vi "Boolean Check Output Result.vi"(9 "Output Value in":cluster{"Name":string, "Variant Data":variant}, 10 "Step Output in":T5, 11 "Execution in":refnum<data-value>) -> (2 "Measure Result out":T1, 3 "Execution out":refnum<data-value>)   [LabVIEW 2015, in "Execution.lvclass"]
uses:
  Execution.lvclass
  Step/STEP_OUTPUT.ctl
  Step/OUTPUT_DATA_TYPE.ctl
  OutputUI/OUTPUT_CHECK_TYPE.ctl
  Step/OUTPUT_VALUE_TYPE.ctl
  STEP_MEASURE_RESULT.ctl
  Step/STEP_STATUS.ctl
  <vilib>/Utility/error.llb/DialogType.ctl
  Get Limit Value Boolean.vi
  Step.lvclass
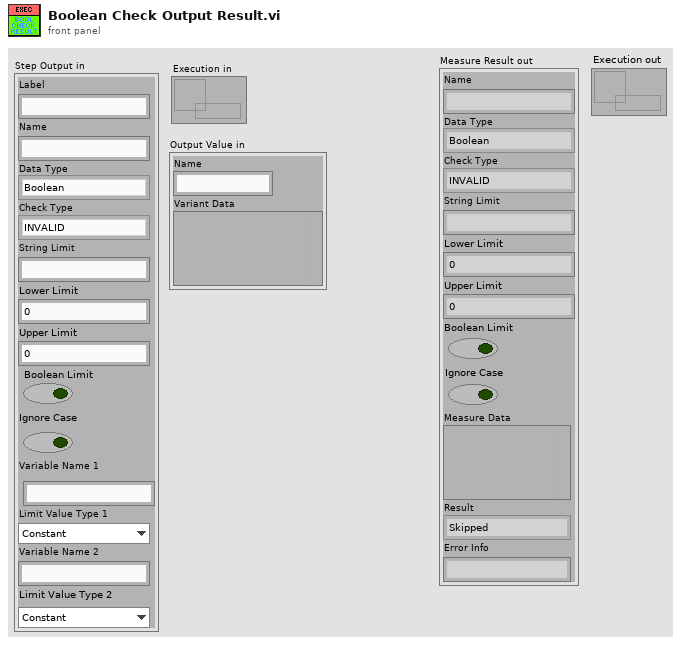
[diagram p1: front panel]
types:
  T1 = typedef "Execution.lvclass/STEP_MEASURE_RESULT.ctl" = cluster{"Name":string, "Data Type":T2, "Check Type":T3, "String Limit":string, "Lower Limit":dbl, "Upper Limit":dbl, "Boolean Limit":bool, "Ignore Case":bool, "Measure Data":variant, "Result":T4, "Error Info":string}
  T2 = typedef "Step.lvclass/OUTPUT_DATA_TYPE.ctl" = enum16{"Boolean", "String", "Numeric", "Other"}
  T3 = typedef "Step.lvclass/OUTPUT_CHECK_TYPE.ctl" = enum16{"INVALID", "DO_NOT_CHECK", "RECORD", "VARIABLE", "EQUAL", "NOT_EQUAL", "STR_CONTAINS", "STR_START_WITH", "STR_END_WITH", "STR_REGEX_MATCH", "NUM_GT", "NUM_LT", "NUM_GE", "NUM_LE", "NUM_RANGE", "NUM_RANGE_BDY"}
  T4 = typedef "Step.lvclass/STEP_STATUS.ctl" = enum16{"Skipped", "Done", "Passed", "Failed", "Error"}
  T5 = typedef "Step.lvclass/STEP_OUTPUT.ctl" = cluster{"Label":string, "Name":string, "Data Type":T2, "Check Type":T3, "String Limit":string, "Lower Limit":dbl, "Upper Limit":dbl, "Boolean Limit":bool, "Ignore Case":bool, "Variable Name 1":string, "Limit Value Type 1":T6, "Variable Name 2":string, "Limit Value Type 2":T6}
  T6 = typedef "Step.lvclass/OUTPUT_VALUE_TYPE.ctl" = enum16{"Constant", "Variable"}
  T7 = typedef "DialogType.ctl" = u16
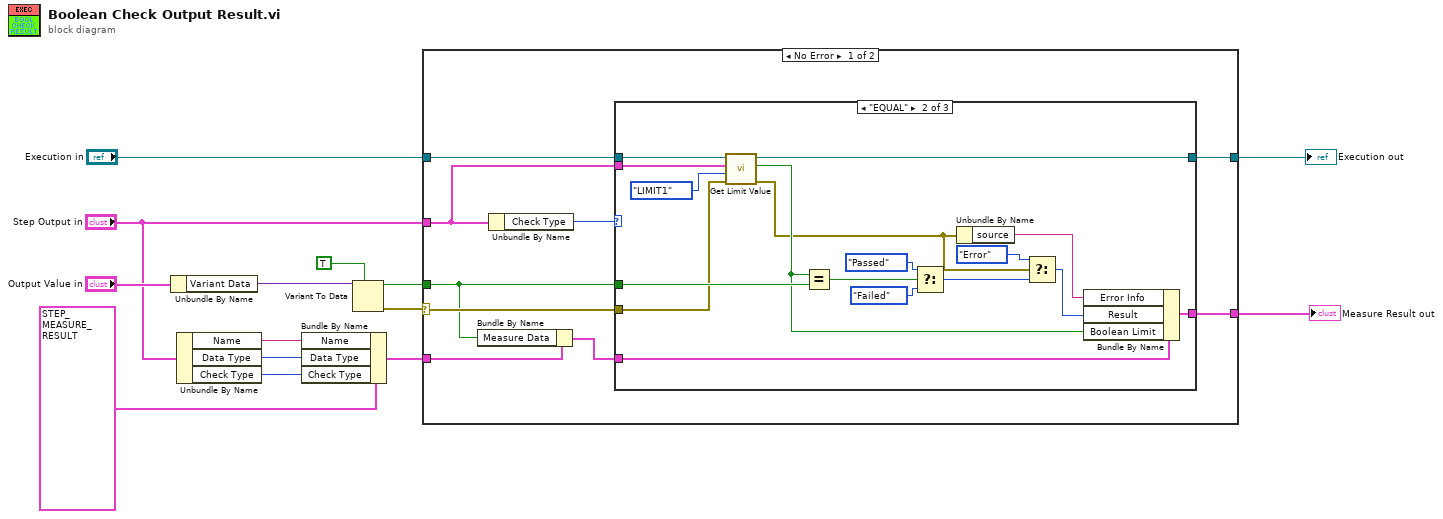
[diagram p0: block diagram]
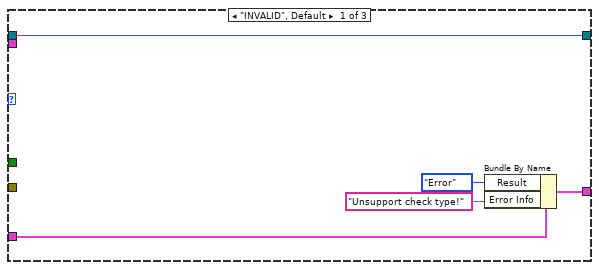
[diagram p2: hidden frame]
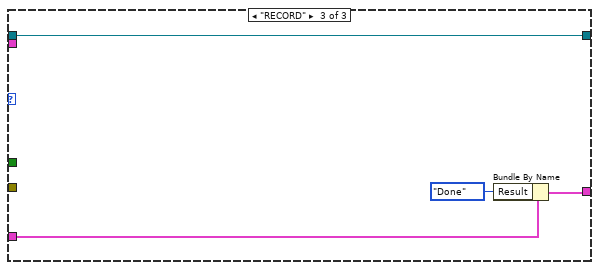
[diagram p3: hidden frame]
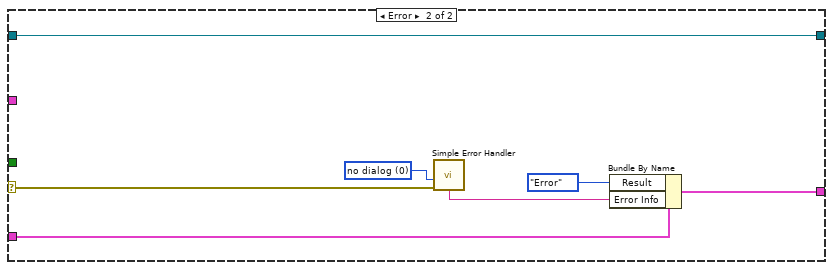
[diagram p4: hidden frame]
diagram:
  n1 = Unbundle By Name("Output Value in") -> ("Variant Data"=w12:variant)
  n2 = Unbundle By Name("Step Output in") -> ("Name"=w5:string, "Data Type"=w4:T2, "Check Type"=w3:T3)
  n3 = Bundle By Name(cluster=T1 {"Name"="", "Data Type"=enum."Boolean", "Check Type"=enum."INVALID", "String Limit"="", "Lower Limit"=0.0, "Upper Limit"=0.0, "Boolean Limit"=FALSE, "Ignore Case"=FALSE, "Measure Data"=variant, "Result"=enum."Skipped", "Error Info"=""} ("Measure Result"), "Name"=w5, "Data Type"=w4, "Check Type"=w3) -> (w2:T1)
  n4 = Variant To Data(type=TRUE, Variant=w12) -> (data=w10:bool, error out=w14:errorcluster)  [unwired: 1 in]
  n5 = case shown="No Error" w14 {
    selector: w14 -> [w19 w55]
    tunnel: "Step Output in" -> [w22 _]
    tunnel: w10 -> [w17 _]
    tunnel: "Execution in" -> [w21 w54]
    tunnel: [w20 w54] -> w8
    tunnel: w2 -> [w18 w53]
    tunnel: [w15 w50] -> w1
    frame No Error {
      n6 = Bundle By Name(cluster=w18, "Measure Data"=w17) -> (w16:T1)
      n7 = Unbundle By Name(w22) -> ("Check Type"=w23:T3)
      n8 = case shown="\"EQUAL\"" w23 {
        tunnel: w22 -> [_ w34 _]
        tunnel: w17 -> [_ w42 _]
        tunnel: w21 -> [w28 w35 w46]
        tunnel: [w28 w29 w46] -> w20
        tunnel: w19 -> [_ w33 _]
        tunnel: w16 -> [w27 w39 w49]
        tunnel: [w24 w36 w48] -> w15
        frame "INVALID", Default {
          n9 = Bundle By Name(cluster=w27, "Result"=STEP_STATUS."Error" ("Status"), "Error Info"="Unsupport check type!") -> (w24:T1)
        }
        frame "EQUAL" {
          n10 = call-poly "Get Limit Value.vi"("error in (no error)"=w33, "Limit"=enum16{"LIMIT1", "LIMIT2"}."LIMIT1", "Step Output in"=w34, "Execution in"=w35) -> ("error out"=w30:errorcluster, "Limit Value"=w31:bool, "Execution out"=w29:refnum<data-value>)  [unwired: 5 in]
          n11 = Equal?(x=w31, y=w42) -> (x = y?=w45:bool)
          n12 = Select(t=STEP_STATUS."Passed" ("Status"), s=w45, f=STEP_STATUS."Failed" ("Status")) -> (s? t:f=w41:T4)
          n13 = Unbundle By Name(w30) -> ("source"=w37:string)
          n14 = Select(t=STEP_STATUS."Error" ("Status"), s=w30, f=w41) -> (s? t:f=w38:T4)
          n15 = Bundle By Name(cluster=w39, "Error Info"=w37, "Result"=w38, "Boolean Limit"=w31) -> (w36:T1)
        }
        frame "RECORD" {
          n16 = Bundle By Name(cluster=w49, "Result"=STEP_STATUS."Done") -> (w48:T1)
        }
      }
    }
    frame Error {
      w56 = T7 0 items=["no dialog", "OK message", "continue or stop message", "OK message + warnings", "continue/stop + warnings"] ("type of dialog (OK msg:1)")
      n17 = call <vilib>:"Simple Error Handler.vi"("type of dialog (OK msg:1)"=w56, "error in (no error)"=w55) -> ("message"=w52:string)  [unwired: 3 in, 4 out]
      n18 = Bundle By Name(cluster=w53, "Result"=STEP_STATUS."Error" ("Status"), "Error Info"=w52) -> (w50:T1)
    }
  }
  "Execution out" <- w8
  "Measure Result out" <- w1
